vi "DrawSite.vi"(4 "y corrector":dbl=1.0, 5 "Color":u32(colorbox)=16711680, 6 "x corrector":dbl=1.0, 7 "Group":string="Mask", 8 "error in (no error)":errorcluster, 9 "Position":cluster{"X":dbl, "Y":dbl, "Z":dbl, "Depth":dbl}, 10 "Scan Properties":T1={"X Size"=512.0, "Y Size"=512.0, "lens"=20.0, "mag"=1.0, "Angle"=0.0}, 11 "Image in":refnum<class "Image.lvclass">) -> (0 "error out":errorcluster, 3 "Image out":refnum<class "Image.lvclass">)   [LabVIEW 2013, in "Image.lvclass"]
uses:
  Image.lvclass
  Image.lvclass/Image.ctl
  <resource>/objmgr/IMAQImage.rc
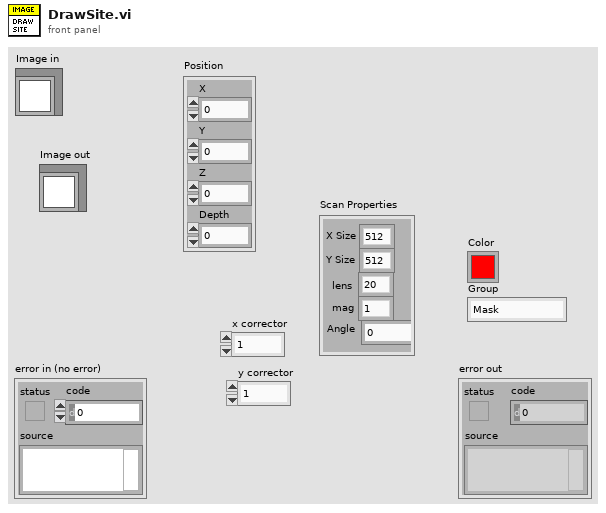
[diagram p1: front panel]
types:
  T1 = cluster{"X Size":dbl, "Y Size":dbl, "lens":dbl, "mag":dbl, "Angle":dbl}
  T2 = typedef "IMAQ Rectangle" = cluster{"Left":i32, "Top":i32, "Right":i32, "Bottom":i32, "Rotation":dbl}
  T3 = typedef "IMAQ Image.ctl" = refnum<image>
  T4 = cluster{"scan_idx":i32, "lens":i32, "mag":dbl, "x":dbl, "y":dbl, "mouse_id":i32, "exp_date":string, "file_name":string, "file_path":path}
  T5 = typedef "ROI Descriptor" = cluster{"Global Rectangle":i32[], "Contours":cluster{"ID":enum32{"External", "Internal"}, "Type":u32, "Coordinates":i32[]}[]}
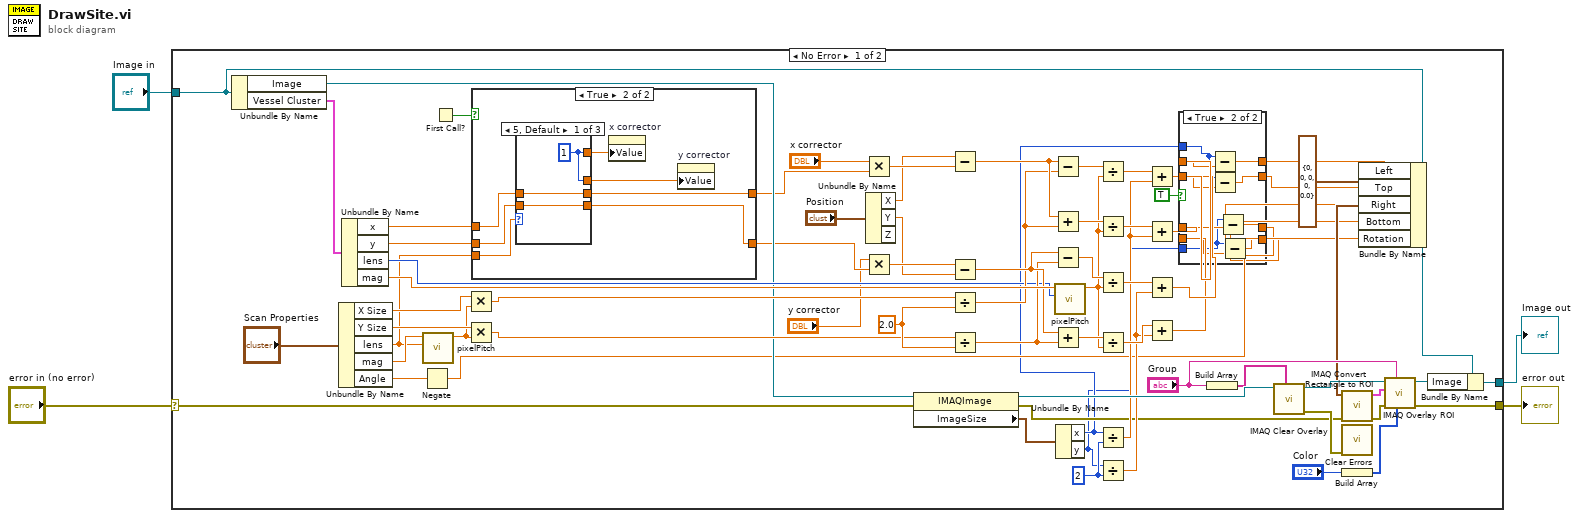
[diagram p0: block diagram]
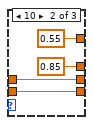
[diagram p4: hidden frame]
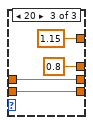
[diagram p5: hidden frame]
diagram:
  n1 = case shown="No Error" "error in (no error)" {
    selector: "error in (no error)" -> [w45 w112]
    tunnel: [w18 w112] -> w3
    tunnel: [w41 w111] -> w1
    tunnel: "Image in" -> [w42 w111]
    frame No Error {
      w66 = 2.0 ("y")
      w76 = 2 ("y")
      n2 = Unbundle By Name(w42) -> ("Image"=w44:T3, "Vessel Cluster"=w43:T4)
      n3 = Unbundle By Name("Scan Properties") -> ("X Size"=w65:dbl, "Y Size"=w64:dbl, "lens"=w46:dbl, "mag"=w71:dbl, "Angle"=w17:dbl)
      n4 = Unbundle By Name(w43) -> ("x"=w48:dbl, "y"=w47:dbl, "lens"=w49:i32, "mag"=w72:dbl)
      n5 = Negate(x=w17) -> (-x=w16:dbl)
      n6 = call "pixelPitch.vi"("Lens"=w46, "Mag"=w71) -> ("PixelPitch"=w63:dbl)  [unwired: 9 in]
      n7 = First Call?() -> (First Call?: T/F=w32:bool)
      n8 = Multiply(x=w65, y=w63) -> (x*y=w61:dbl)
      n9 = Multiply(x=w64, y=w63) -> (x*y=w60:dbl)
      n10 = case shown="True" w32 {
        tunnel: w48 -> [w92 w99]
        tunnel: w47 -> [w91 w98]
        tunnel: w46 -> [_ w97]
        tunnel: [w92 w96] -> w38
        tunnel: [w91 w95] -> w34
        frame False {
        }
        frame True {
          n11 = case shown="5, Default" w97 {
            tunnel: w99 -> [w102 w106 w110]
            tunnel: [w102 w106 w110] -> w96
            tunnel: w98 -> [w101 w104 w109]
            tunnel: [w101 w104 w109] -> w95
            tunnel: [w100 0.55 ("x") 1.15] -> w94
            tunnel: [w100 0.85 ("y") 0.8] -> w93
            frame 5, Default {
              w100 = 1
            }
            frame 10 {
            }
            frame 20 {
            }
          }
          n12 = property on="x corrector" class="DigNum (strict)"("Value"=w94) -> ()  [unwired: 2 in, 2 out]
          n13 = property on="y corrector" class="DigNum (strict)"("Value"=w93) -> ()  [unwired: 2 in, 2 out]
        }
      }
      n14 = Multiply(x="x corrector", y=w38) -> (x*y=w37:dbl)
      n15 = Multiply(x="y corrector", y=w34) -> (x*y=w35:dbl)
      n16 = Unbundle By Name("Position") -> ("X"=w30:dbl, "Y"=w29:dbl)  [unwired: 1 out]
      n17 = property class="IMAQImage"(reference=w44, error in=w45) -> (reference out=w74:T3, error out=w20:errorcluster, "ImageSize"=w75:cluster{"x":i32, "y":i32})
      n18 = Subtract(x=w30, y=w37) -> (x-y=w52:dbl)
      n19 = Subtract(x=w35, y=w29) -> (x-y=w53:dbl)
      n20 = Divide(x=w61, y=w66) -> (x/y=w51:dbl)
      n21 = Divide(x=w60, y=w66) -> (x/y=w50:dbl)
      n22 = Subtract(x=w52, y=w51) -> (x-y=w67:dbl)
      n23 = Add(x=w52, y=w51) -> (x+y=w70:dbl)
      n24 = Subtract(x=w53, y=w50) -> (x-y=w68:dbl)
      n25 = Add(x=w53, y=w50) -> (x+y=w69:dbl)
      n26 = call "pixelPitch.vi"("Lens"=w49, "Mag"=w72) -> ("PixelPitch"=w62:dbl)  [unwired: 9 in]
      n27 = Unbundle By Name(w75) -> ("x"=w7:i32, "y"=w6:i32)
      n28 = Divide(x=w67, y=w62) -> (x/y=w59:dbl)
      n29 = Divide(x=w70, y=w62) -> (x/y=w57:dbl)
      n30 = Divide(x=w68, y=w62) -> (x/y=w58:dbl)
      n31 = Divide(x=w69, y=w62) -> (x/y=w56:dbl)
      n32 = Divide(x=w7, y=w76) -> (x/y=w55:dbl)
      n33 = Divide(x=w6, y=w76) -> (x/y=w54:dbl)
      n34 = Add(x=w59, y=w55) -> (x+y=w15:dbl)
      n35 = Add(x=w57, y=w55) -> (x+y=w13:dbl)
      n36 = Add(x=w58, y=w54) -> (x+y=w14:dbl)
      n37 = Add(x=w56, y=w54) -> (x+y=w12:dbl)
      n38 = case shown="True" TRUE {
        tunnel: w15 -> [w80 w86]
        tunnel: w14 -> [w79 w85]
        tunnel: w13 -> [w78 w84]
        tunnel: w12 -> [w77 w83]
        tunnel: [w80 w90] -> w11
        tunnel: [w79 w89] -> w10
        tunnel: [w78 w88] -> w9
        tunnel: [w77 w87] -> w8
        tunnel: w7 -> [_ w82]
        tunnel: w6 -> [_ w81]
        frame False {
        }
        frame True {
          n39 = Subtract(x=w82, y=w86) -> (x-y=w90:dbl)
          n40 = Subtract(x=w82, y=w85) -> (x-y=w89:dbl)
          n41 = Subtract(x=w81, y=w84) -> (x-y=w88:dbl)
          n42 = Subtract(x=w81, y=w83) -> (x-y=w87:dbl)
        }
      }
      n43 = Build Array("Group") -> (w40:string[])
      n44 = call "IMAQ Clear Overlay"("Groups"=w40, "Image"=w74) -> ("error out"=w39:errorcluster, "Image Out"=w27:T3)  [unwired: 1 in, 7 out]
      n45 = call <vilib>:"Clear Errors.vi"("error in (no error)"=w39) -> ()  [unwired: 6 in, 1 out]
      n46 = Build Array("Color") -> (w21:u32[])
      n47 = Bundle By Name(cluster=T2 {"Left"=0, "Top"=0, "Right"=0, "Bottom"=0, "Rotation"=0.0} ("Rectangle"), "Left"=w11, "Top"=w10, "Right"=w9, "Bottom"=w8, "Rotation"=w16) -> (w23:T2)
      n48 = call "IMAQ Convert Rectangle to ROI"("error in (no error)"=w20, "Rectangle"=w23) -> ("error out"=w19:errorcluster, "ROI Descriptor"=w28:T5)  [unwired: 7 in]
      n49 = call "IMAQ Overlay ROI"("Colors (Green)"=w21, "Group"="Group", "error in (no error)"=w19, "ROI Descriptor"=w28, "Image"=w27) -> ("error out"=w18:errorcluster, "Image Out"=w25:T3)  [unwired: 5 in]
      n50 = Bundle By Name(cluster=w42, "Image"=w25) -> (w41:refnum<class "Image.lvclass">)
    }
    frame Error {
    }
  }
  "error out" <- w3
  "Image out" <- w1
